vi "clone.vi"(0 "reference":refnum<class "MultiLineString.lvclass">, 5 "error in (no error)":errorcluster) -> (14 "reference out":refnum<class "MultiLineString.lvclass">, 15 "clonedMultiLineString":refnum<class "MultiLineString.lvclass">, 19 "error out":errorcluster)   [LabVIEW 2020, in "MultiLineString.lvclass"]
doc: "public Object clone()"
uses:
  <resource>/Framework/Providers/Open_GDS/UML/MultiLineString_class/MultiLineString.lvclass
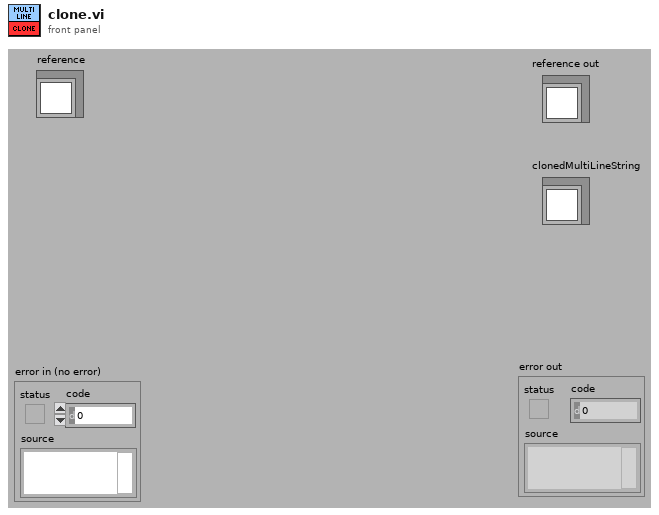
[diagram p1: front panel]
types:
  T1 = typedef "MultiLineString.lvclass/ObjectAttributes.ctl" = cluster{"GAP":i32, "text":string, "justification":T2, "size":T3, "underlined":bool}
  T2 = typedef "MultiLineString.lvclass/JustificationType.ctl" = enum16{"LEFT", "CENTER", "RIGHT"}
  T3 = typedef "MultiLineString.lvclass/SizeType.ctl" = enum16{"LARGE", "NORMAL", "SMALL"}
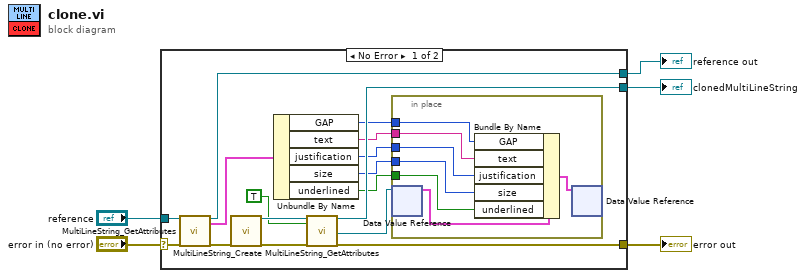
[diagram p0: block diagram]
diagram:
  n1 = case shown="No Error" "error in (no error)" {
    selector: "error in (no error)" -> [w14 w29]
    tunnel: "reference" -> [w21 w30]
    tunnel: [w20 w29] -> w4
    tunnel: [w19 w30] -> w3
    tunnel: [w18 _] -> w1
    frame No Error {
      n2 = call <resource>:"MultiLineString_GetAttributes.vi"("reference in"=w21, "error in (no error)"=w14) -> ("reference out"=w19:refnum<class "MultiLineString.lvclass">, "Data"=w12:T1, "error out"=w15:errorcluster)  [unwired: 1 in, 14 out]
      n3 = call <resource>:"MultiLineString_Create.vi"("error in (no error)"=w15) -> ("reference out"=w17:refnum<class "MultiLineString.lvclass">, "error out"=w16:errorcluster)  [unwired: 2 in, 15 out]
      n4 = Unbundle By Name(w12) -> ("GAP"=w10:i32, "text"=w9:string, "justification"=w8:T2, "size"=w7:T3, "underlined"=w6:bool)
      n5 = call <resource>:"MultiLineString_GetAttributes.vi"("reference in"=w17, "OnlyGetDvrReference(False)"=TRUE, "error in (no error)"=w16) -> ("reference out"=w18:refnum<class "MultiLineString.lvclass">, "DataRef"=w11:refnum<data-value>, "error out"=w20:errorcluster)  [unwired: 13 in, 1 out]
      n6 = in-place {
        in-place-border: w10 -> [w27]
        in-place-border: w9 -> [w26]
        in-place-border: w8 -> [w25]
        in-place-border: w7 -> [w24]
        in-place-border: w6 -> [w23]
        n7 = in-place-dvr #1(w11) -> (w28:T1)  [unwired: 1 out]
        n8 = Bundle By Name(cluster=w28, "GAP"=w27, "text"=w26, "justification"=w25, "size"=w24, "underlined"=w23) -> (w22:T1)
        n9 = in-place-dvr #1(w22) -> ()  [unwired: 2 out]
      }
    }
    frame Error {
    }
  }
  "reference out" <- w3
  "error out" <- w4
  "clonedMultiLineString" <- w1
